vi "EmptyStr2YYYY-MM-DD_hh-mm-ss_.vi"(1 "file_name":string caption="Input Name :") -> (0 "OutputName":string)   [LabVIEW 2018]
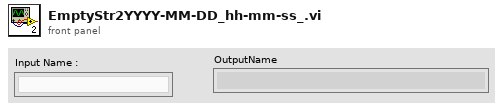
[diagram p1: front panel]
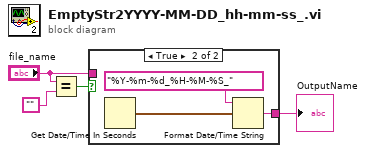
[diagram p0: block diagram]
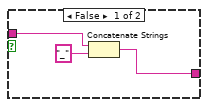
[diagram p2: hidden frame]
diagram:
  n1 = Equal?(x="file_name", y="") -> (x = y?=w3:bool)
  n2 = case shown="True" w3 {
    tunnel: "file_name" -> [w7 _]
    tunnel: [w5 w8] -> w1
    frame False {
      n3 = Concatenate Strings(w7, "_" ("string")) -> (w5:string)
    }
    frame True {
      n4 = Get Date/Time In Seconds() -> (seconds since 1Jan1904=w9:timestamp)
      n5 = Format Date/Time String(time format string (%c)="%Y-%m-%d_%H-%M-%S_", seconds (now)=w9) -> (date/time string=w8:string)  [unwired: 1 in]
    }
  }
  "OutputName" <- w1
